vi "Read Frequency Target.vi"(8 "error in (no error)":errorcluster, 11 "FEA_Model in":refnum<class "FEA_Model.lvclass">) -> (0 "error out":errorcluster, 2 "Frequency Target":dbl, 3 "FEA_Model out":refnum<class "FEA_Model.lvclass">)   [LabVIEW 2021, in "FEA_Model.lvclass"]
uses:
  FEA_Model.lvclass
  FEA_Model.lvclass/FEA_Model.ctl
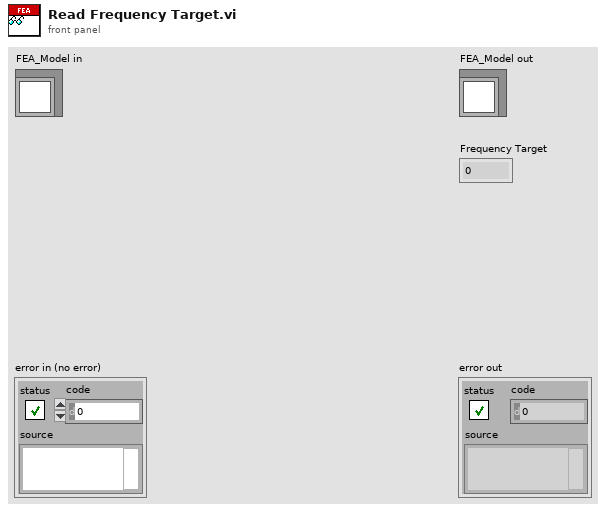
[diagram p1: front panel]
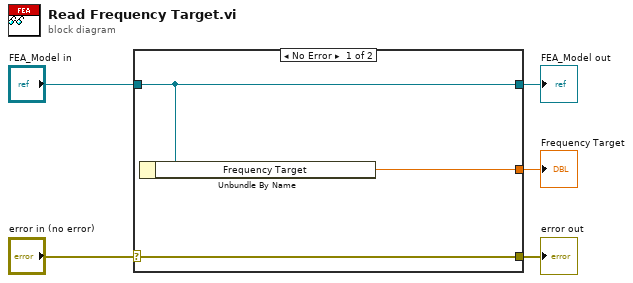
[diagram p0: block diagram]
diagram:
  n1 = case shown="No Error" "error in (no error)" {
    selector: "error in (no error)" -> [w8 w9]
    tunnel: [w8 w9] -> w4
    tunnel: [w7 w10] -> w2
    tunnel: "FEA_Model in" -> [w7 w10]
    tunnel: [w6 _] -> w1
    frame No Error {
      n2 = Unbundle By Name(w7) -> ("Frequency Target"=w6:dbl)
    }
    frame Error {
    }
  }
  "error out" <- w4
  "FEA_Model out" <- w2
  "Frequency Target" <- w1
